vi "Read Repeats.vi"(8 "error in (no error)":errorcluster, 11 "RampProgramModel in":refnum<class "RampProgramModel.lvclass">) -> (0 "error out":errorcluster, 2 "Repeats":u32, 3 "RampProgramModel out":refnum<class "RampProgramModel.lvclass">)   [LabVIEW 2013, in "RampProgramModel.lvclass"]
uses:
  RampProgramModel.lvclass
  RampProgramModel.lvclass/RampProgramModel.ctl
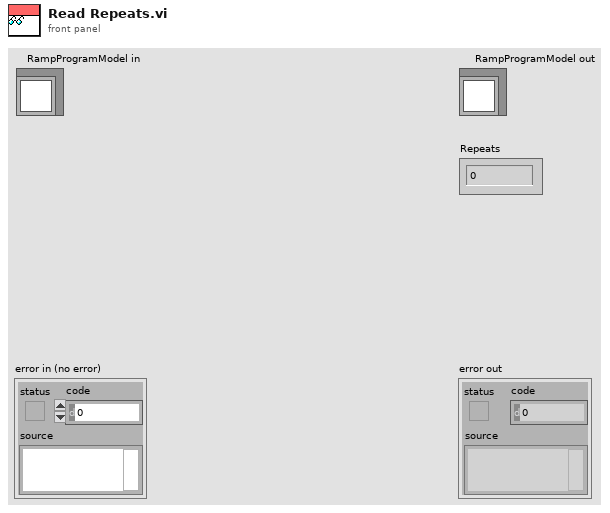
[diagram p1: front panel]
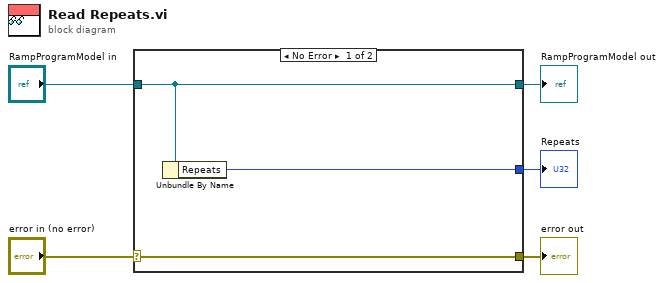
[diagram p0: block diagram]
diagram:
  n1 = case shown="No Error" "error in (no error)" {
    selector: "error in (no error)" -> [w8 w9]
    tunnel: [w8 w9] -> w4
    tunnel: [w7 w10] -> w2
    tunnel: "RampProgramModel in" -> [w7 w10]
    tunnel: [w6 _] -> w1
    frame No Error {
      n2 = Unbundle By Name(w7) -> ("Repeats"=w6:u32)
    }
    frame Error {
    }
  }
  "error out" <- w4
  "RampProgramModel out" <- w2
  "Repeats" <- w1
